vi "FIFO_Host.vi"() -> ()   [LabVIEW 2022 SP3]
uses:
  <vilib>/rvi/interface/nirviMethod/nirviMethod.xnode
  <vilib>/rvi/errors/niLvFpgaMergeErrorWithErrorCode.vi
  <vilib>/rvi/interface/nirviOpenFPGA/nirviOpenFPGA.xnode
  <vilib>/FPGAPlugInAG/Dynamic/niLvFpga_Reset_Dynamic.vi
  <vilib>/FPGAPlugInAG/Dynamic/niLvFpga_Run_Dynamic.vi
  <vilib>/rvi/interface/nirviCloseFPGA/nirviCloseFPGA.xnode
  FPGA Bitfiles/fifoproject_FPGATarget_FIFOTarget_lWIJW4U0KnI.lvbitx
  <vilib>/FPGAPlugInAG/cRIO-9035/niLvFpga_Open_cRIO-9035.vi
  <vilib>/rvi/interface/common/dynamic/niFpgaDynamicAddResources.vi
  <vilib>/FPGAPlugInAG/Dynamic/niLvFpga_Close_Dynamic.vi
  <vilib>/FPGAPlugInAG/Dynamic/niLvFpga_WriteFifo_Dynamic.vi
  <vilib>/FPGAPlugInAG/Dynamic/niLvFpga_ReadFifo_Dynamic.vi
panel:
  out "Numeric":i32
  out "Controlled Force":sgl[](graph)
  out "Uncontrolled Displacement":dynamicdata(graph)
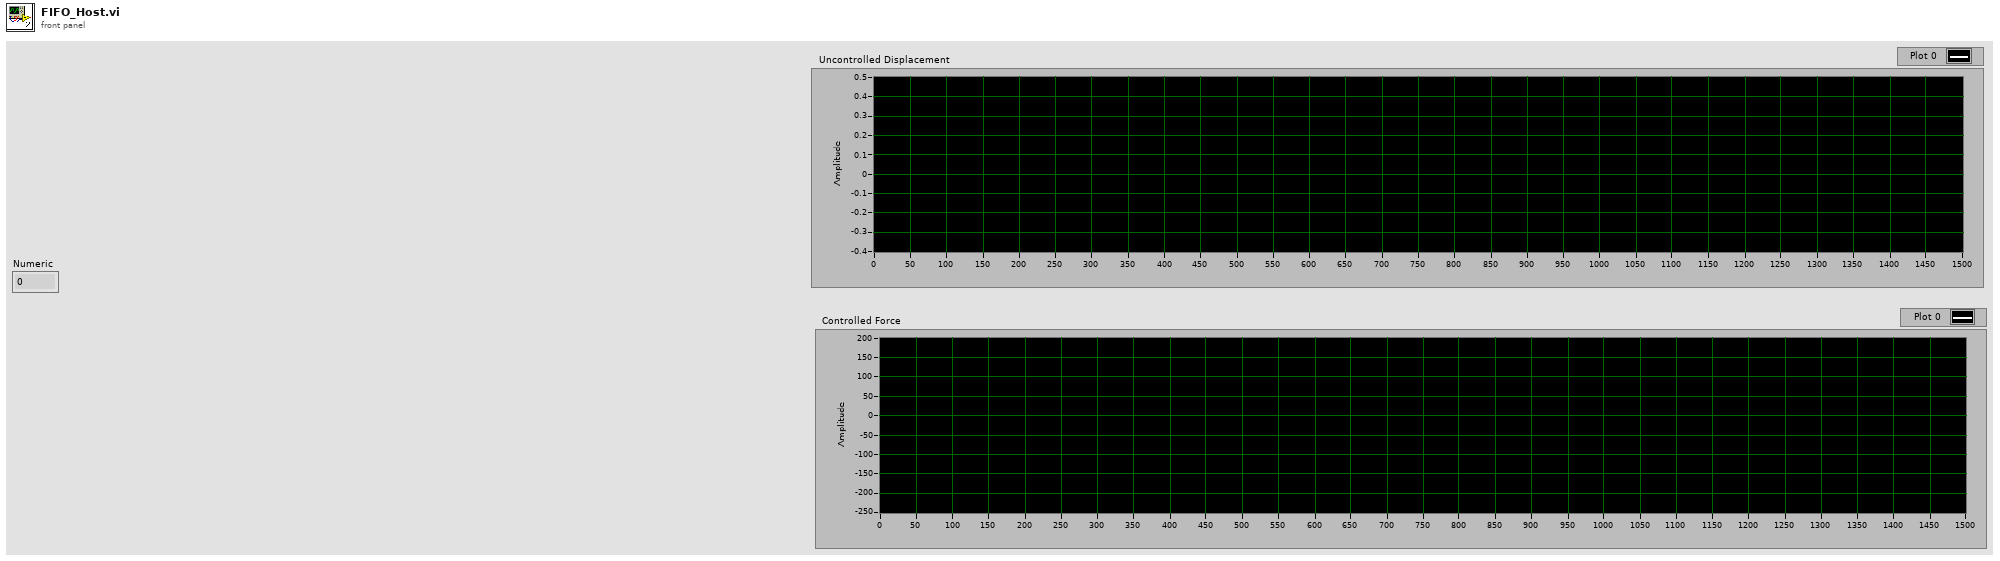
[diagram p1: front panel]
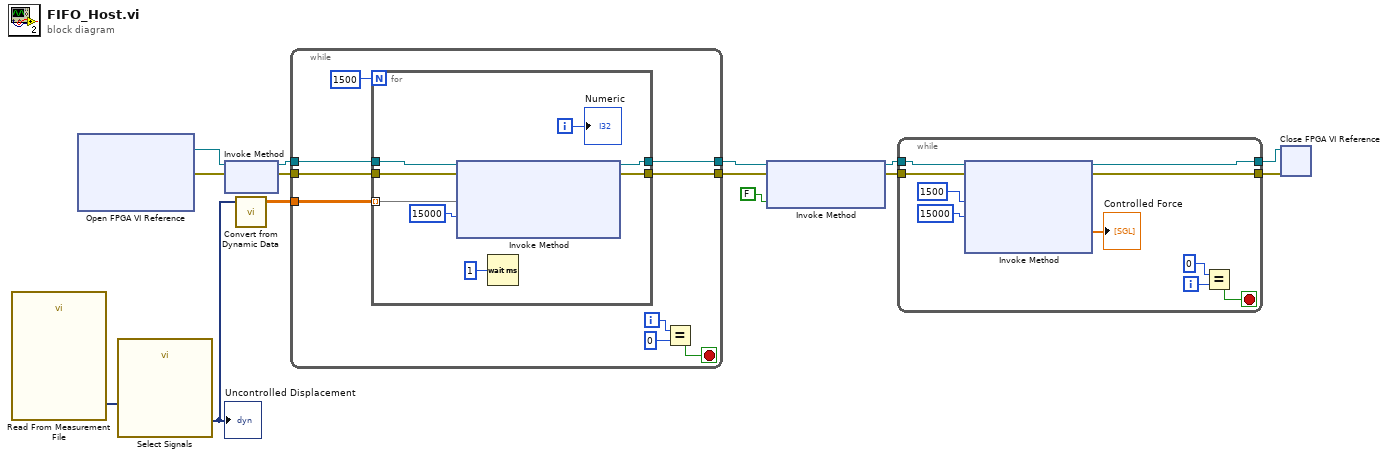
[diagram p0: block diagram]
diagram:
  n1 = call "Read From Measurement File"() -> ("Signals"=w14:dynamicdata)  [unwired: 6 in, 5 out]
  n2 = xnode "Open FPGA VI Reference"() -> ("FPGA VI Reference Out"=w11:refnum<k20>, "error out"=w5:errorcluster)  [unwired: 2 in]
  n3 = call "Select Signals"("Signals"=w14) -> ("Signal Out"=w13:dynamicdata)  [unwired: 9 in, 1 out]
  "Uncontrolled Displacement" <- w13
  n4 = xnode "Invoke Method"("FPGA VI Reference In"=w11, "error in"=w5) -> ("FPGA VI Reference Out"=w10:refnum<k20>, "error out"=w4:errorcluster)
  n5 = call "Convert from Dynamic Data"("Dynamic Data Type"=w13) -> ("Array"=w12:dbl[][])  [unwired: 3 in]
  n6 = while {
    tunnel: w12 -> [w22]
    tunnel: w10 -> [w21]
    tunnel: [w19] -> w9
    tunnel: w4 -> [w16]
    tunnel: [w15] -> w3
    i -> [w17]
    stop <- w20 stop-if-true
    n7 = for {
      N: 1500 -> [_]
      tunnel: w22 -> [w28] mode=indexing
      tunnel: w21 -> [w29]
      tunnel: [w27] -> w19
      tunnel: w16 -> [w25]
      tunnel: [w24] -> w15
      i -> [w26]
      n8 = xnode "Invoke Method"("FPGA VI Reference In"=w29, "error in"=w25, "Data"=w28, "Timeout (ms)"=15000) -> ("FPGA VI Reference Out"=w27:refnum<k20>, "error out"=w24:errorcluster)  [unwired: 1 out]
      n9 = Wait (ms)(milliseconds to wait=u32 1) -> ()  [unwired: 1 out]
      "Numeric" <- w26
    }
    n10 = Equal?(x=w17, y=u32 0) -> (x = y?=w20:bool)
  }
  n11 = xnode "Invoke Method"("FPGA VI Reference In"=w9, "error in"=w3, "Wait Until Done (F)"=FALSE) -> ("FPGA VI Reference Out"=w8:refnum<k20>, "error out"=w2:errorcluster)
  n12 = while {
    tunnel: [w40] -> w6
    tunnel: w8 -> [w38]
    tunnel: w2 -> [w33]
    tunnel: [w32] -> w1
    i -> [w37]
    stop <- w35 stop-if-true
    n13 = xnode "Invoke Method"("FPGA VI Reference In"=w38, "error in"=w33, "Number of Elements"=u32 1500, "Timeout (ms)"=15000) -> ("FPGA VI Reference Out"=w40:refnum<k20>, "error out"=w32:errorcluster, "Data"=→"Controlled Force":sgl[])  [unwired: 1 out]
    n14 = Equal?(x=0, y=w37) -> (x = y?=w35:bool)
  }
  n15 = xnode "Close FPGA VI Reference"("FPGA VI Reference In"=w6, "error in"=w1) -> ()  [unwired: 1 out]
